vi "PositionControl.vi"(6 "ConsecutiveTargets":i32, 7 "ErrorDeadband":dbl, 8 "MaxOutput":dbl, 9 "MinOutput":dbl, 10 "ErrorThreshold":dbl, 11 "Error":dbl) -> (0 "UnfilteredOnTarget":bool, 2 "OnTarget":bool, 3 "OutputValue":dbl)   [LabVIEW 2023]
doc: "Calculates an output to help reach a target based on the current error and calibration parameters.\n\nInputs:\n-- ErrorDeadband -- Double -- The Deadband or range of values that will be considered to be \"ontarget\" --\n-- Error -- Double -- The Error of your current value from the target value (Target - Value) --\n-- MinOutput -- Double -- The minimum output the system is capable of outputting -- \n-- MaxOutput -- Double -- The maximum output the system is capableof outputting-\n-- ConsecutiveTargets -- Boolean -- The number of times you must remain on target to confidently be on target --\n\nOutputs:\n-- OutputValue -- Double -- The output value desired to help reach your target --\n-- OnTarget -- Boolean -- True if you are confidently on target --\n-- UnfilteredOnTarget -- Boolean -- True if position control thinks you are on target for 1 loop. NOT RECOMENDED FOR USE IN ROBOT CODE, only meant for debugging --"
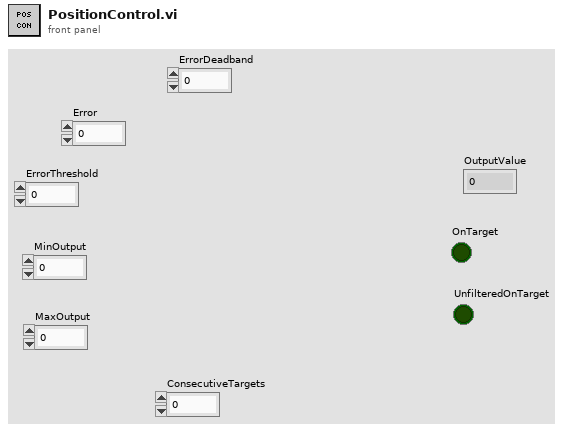
[diagram p1: front panel]
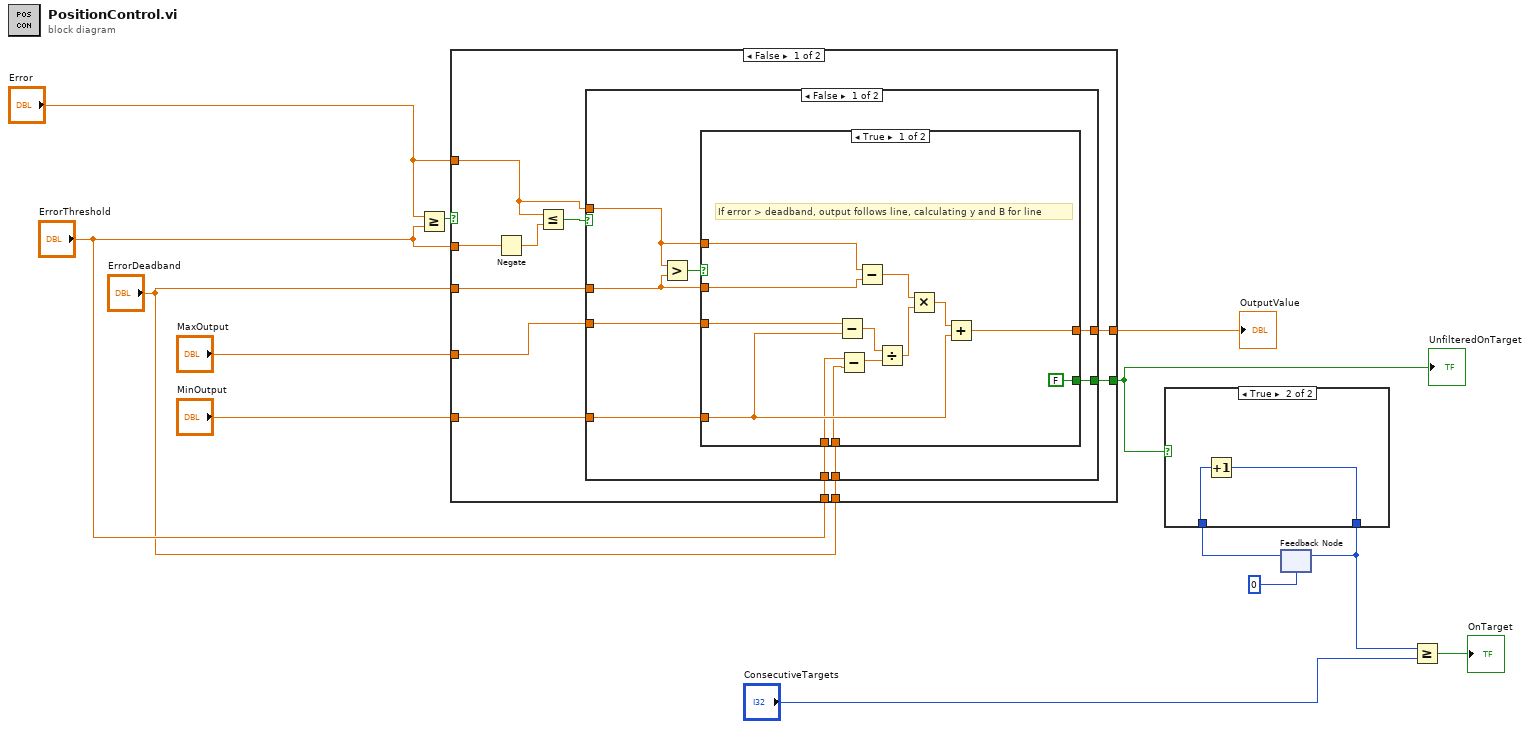
[diagram p0: block diagram]
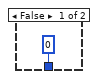
[diagram p2: hidden frame]
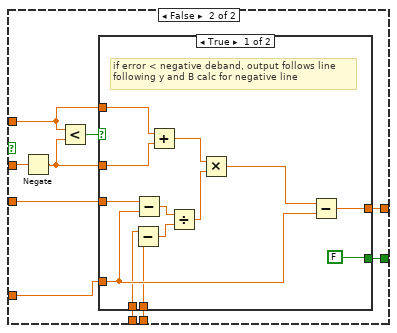
[diagram p3: hidden frame]
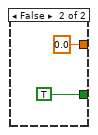
[diagram p4: hidden frame]
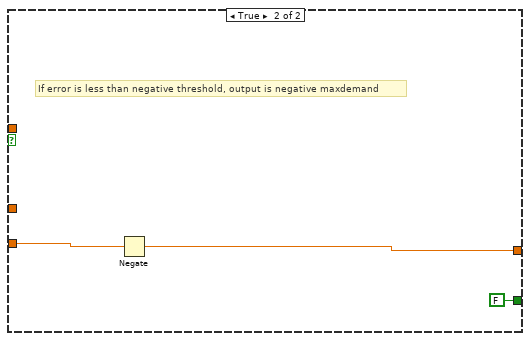
[diagram p5: hidden frame]
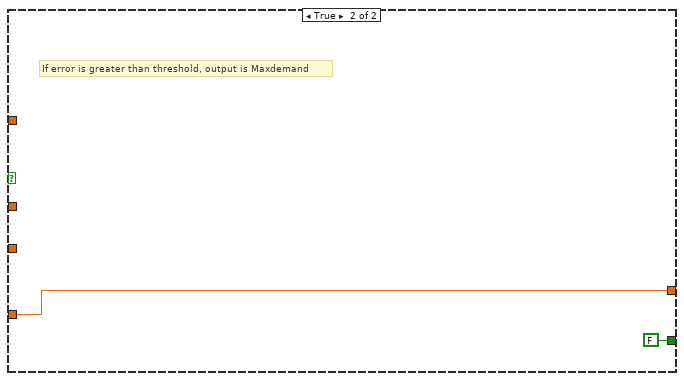
[diagram p6: hidden frame]
diagram:
  n1 = Greater Or Equal?(x="Error", y="ErrorThreshold") -> (x >= y?=w11:bool)
  n2 = case shown="False" w11 {
    tunnel: [w20 w76] -> w13
    tunnel: "MaxOutput" -> [w21 w76]
    tunnel: "Error" -> [w19 _]
    tunnel: "ErrorThreshold" -> [w22 _]
    tunnel: "ErrorDeadband" -> [w18 _]
    tunnel: "MinOutput" -> [w17 _]
    tunnel: "ErrorThreshold" -> [w16 _]
    tunnel: "ErrorDeadband" -> [w15 _]
    tunnel: [w14 FALSE] -> w3
    frame False {
      n3 = Negate(x=w22) -> (-x=w23:dbl)
      n4 = Less Or Equal?(x=w19, y=w23) -> (x <= y?=w24:bool)
      n5 = case shown="False" w24 {
        tunnel: w21 -> [w28 w74]
        tunnel: [w32 w73] -> w20
        tunnel: w19 -> [w30 _]
        tunnel: w18 -> [w29 _]
        tunnel: w17 -> [w31 _]
        tunnel: w16 -> [w27 _]
        tunnel: w15 -> [w26 _]
        tunnel: [w25 FALSE] -> w14
        frame False {
          n6 = Greater?(x=w30, y=w29) -> (0:w33:bool)
          n7 = case shown="True" w33 {
            tunnel: [w46 w56] -> w32
            tunnel: w31 -> [w38 w52]
            tunnel: w30 -> [w45 w54]
            tunnel: w29 -> [w44 w48]
            tunnel: w28 -> [w39 w53]
            tunnel: w27 -> [w37 w51]
            tunnel: w26 -> [w36 w50]
            tunnel: [FALSE w49] -> w25
            frame True {
              # "If error > deadband, output follows line, calculating y and B for line"
              n8 = Subtract(x=w39, y=w38) -> (x-y=w41:dbl)
              n9 = Subtract(x=w37, y=w36) -> (x-y=w40:dbl)
              n10 = Subtract(x=w45, y=w44) -> (x-y=w43:dbl)
              n11 = Divide(x=w41, y=w40) -> (x/y=w42:dbl)
              n12 = Multiply(x=w43, y=w42) -> (x*y=w35:dbl)
              n13 = Add(x=w35, y=w38) -> (x+y=w46:dbl)
            }
            frame False {
              n14 = Negate(x=w48) -> (-x=w47:dbl)
              n15 = Less?(x=w54, y=w47) -> (x < y?=w55:bool)
              n16 = case shown="True" w55 {
                tunnel: [w69 0.0] -> w56
                tunnel: w52 -> [w61 _]
                tunnel: w54 -> [w68 _]
                tunnel: w47 -> [w67 _]
                tunnel: w53 -> [w62 _]
                tunnel: w51 -> [w60 _]
                tunnel: w50 -> [w59 _]
                tunnel: [FALSE TRUE] -> w49
                frame True {
                  # "if error < negative deband, output follows line\nfollowing y and B calc for negative line"
                  n17 = Subtract(x=w60, y=w59) -> (x-y=w63:dbl)
                  n18 = Subtract(x=w62, y=w61) -> (x-y=w64:dbl)
                  n19 = Add(x=w68, y=w67) -> (x+y=w66:dbl)
                  n20 = Divide(x=w64, y=w63) -> (x/y=w65:dbl)
                  n21 = Multiply(x=w66, y=w65) -> (x*y=w58:dbl)
                  n22 = Subtract(x=w58, y=w61) -> (x-y=w69:dbl)
                }
                frame False {
                }
              }
            }
          }
        }
        frame True {
          # "If error is less than negative threshold, output is negative maxdemand"
          n23 = Negate(x=w74) -> (-x=w73:dbl)
        }
      }
    }
    frame True {
      # "If error is greater than threshold, output is Maxdemand"
    }
  }
  "OutputValue" <- w13
  "UnfilteredOnTarget" <- w3
  n24 = feedback #1(0) -> (w2:i32)
  n25 = case shown="True" w3 {
    tunnel: w2 -> [_ w79]
    tunnel: [0 w78] -> w1
    frame False {
    }
    frame True {
      n26 = Increment(x=w79) -> (x+1=w78:i32)
    }
  }
  n27 = feedback-in #1(w1) -> ()
  n28 = Greater Or Equal?(x=w1, y="ConsecutiveTargets") -> (x >= y?=→"OnTarget":bool)
